vi "turn.vi"(8 "out of gas warning":bool, 9 "Gear":T1(ring), 10 "Cluster":T2, 11 "Array":T3[](array[typedef]) {"Data" format="%.0x"}) -> (3 "Array 2":T3[](array[typedef]) {"Data" format="%.0x"})   [LabVIEW 2021, in "uCanDriver.lvlib" / "uCAN.lvclass"]
uses:
  uCAN.lvclass
  typedefs/frame.ctl
  typedefs/control leds.ctl
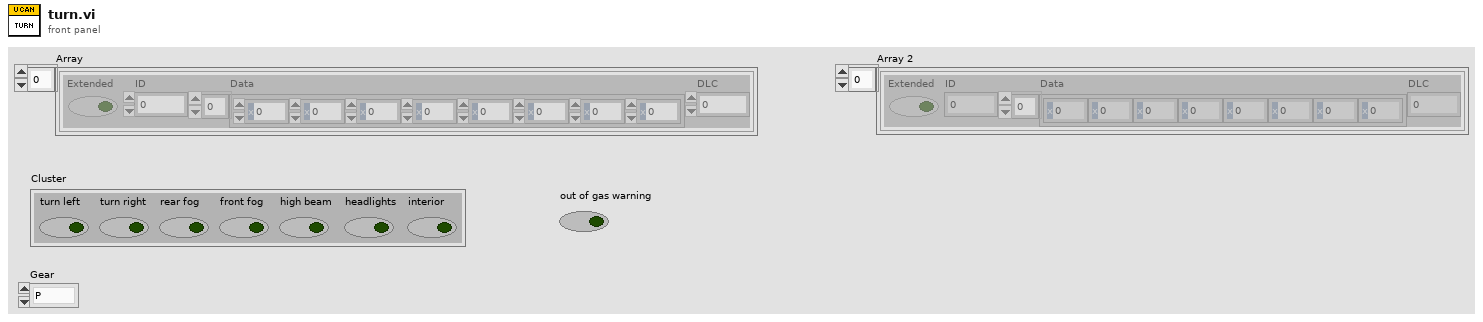
[diagram p1: front panel]
types:
  T1 = enum16{"P", "R", "N", "-", "6", "5", "4", "3", "2", "1", ""}
  T2 = typedef "control leds.ctl" = cluster{"turn left":bool, "turn right":bool, "rear fog":bool, "front fog":bool, "high beam":bool, "headlights":bool, "interior":bool}
  T3 = typedef "uCanDriver.lvlib/uCAN.lvclass/frame.ctl" = cluster{"Extended":bool, "ID":u32, "Data":u8[], "DLC":u8}
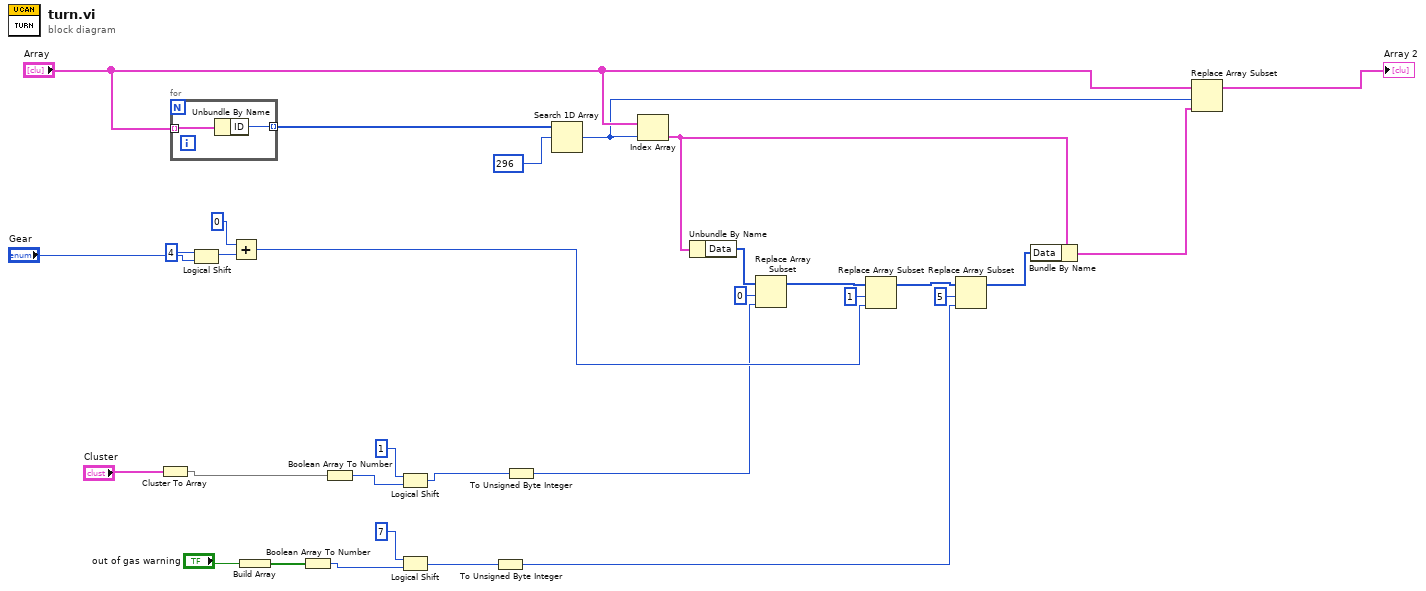
[diagram p0: block diagram]
diagram:
  n1 = Cluster To Array(cluster="Cluster") -> (array=w10:bool[])
  n2 = for {
    tunnel: "Array" -> [w33] mode=indexing
    tunnel: [w32] -> w29 mode=indexing
    n3 = Unbundle By Name(w33) -> ("ID"=w32:u32)
  }
  n4 = Logical Shift(y=i16 4, x="Gear") -> (x << y=w18:u32)
  n5 = Add(x=u32 0, y=w18) -> (x+y=w16:u32)
  n6 = Build Array("out of gas warning") -> (w4:bool[])
  n7 = Boolean Array To Number(Boolean array=w4) -> (number=w3:u32)
  n8 = Boolean Array To Number(Boolean array=w10) -> (number=w13:u32)
  n9 = Logical Shift(y=i16 1, x=w13) -> (x << y=w12:u32)
  n10 = Logical Shift(y=i16 7, x=w3) -> (x << y=w2:u32)
  n11 = To Unsigned Byte Integer(number=w2) -> (unsigned 8bit integer=w1:u8)
  n12 = To Unsigned Byte Integer(number=w12) -> (unsigned 8bit integer=w15:u8)
  n13 = Search 1D Array(1D array=w29, element=u32 296) -> (index of element=w27:i32)  [unwired: 1 in]
  n14 = Index Array(array="Array", index=w27) -> (element=w31:T3)
  n15 = Unbundle By Name(w31) -> ("Data"=w24:u8[])
  n16 = Replace Array Subset(array=w24, new element=w15, index=0) -> (w21:u8[])
  n17 = Replace Array Subset(array=w21, new element=w16, index=1) -> (w8:u8[])
  n18 = Replace Array Subset(array=w8, new element=w1, index=5) -> (w7:u8[])
  n19 = Bundle By Name(cluster=w31, "Data"=w7) -> (w25:T3)
  n20 = Replace Array Subset(array="Array", new element=w25, index=w27) -> (→"Array 2":T3[])
